vi "Alpha_Beta_prunning.vi"(0 "Game":i32[][](array[numeric]), 1 "Active Turn":i32=1, 2 "Depth":i32, 5 "NextTurn":i32=1) -> (10 "Win":bool, 11 "GameOver":bool, 14 "Score":i32, 15 "Next Move":cluster{"Row":i32, "Col":i32}, 17 "Scores":i32[](array[numeric]), 18 "Moves":cluster{"Row":i32, "Col":i32}[](array[cluster]))   [LabVIEW 2017]
panel:
  out "Array (Ausgang)":i32[][](array[numeric])
  in  "Max Depth (7)":i32=7 min=7 max=23
  # "3x3 Felder Max Depth 7\n4*4 Felder Max Depth 15\n5*5 Felder Max Depth 23"
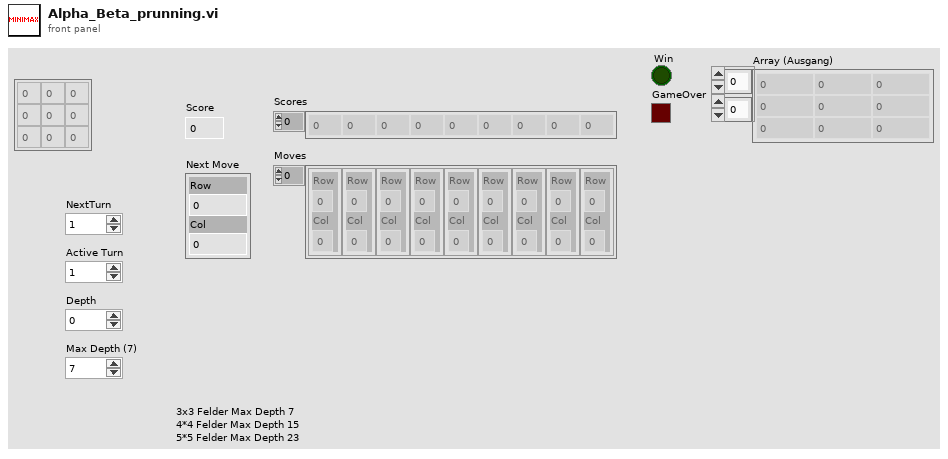
[diagram p1: front panel]
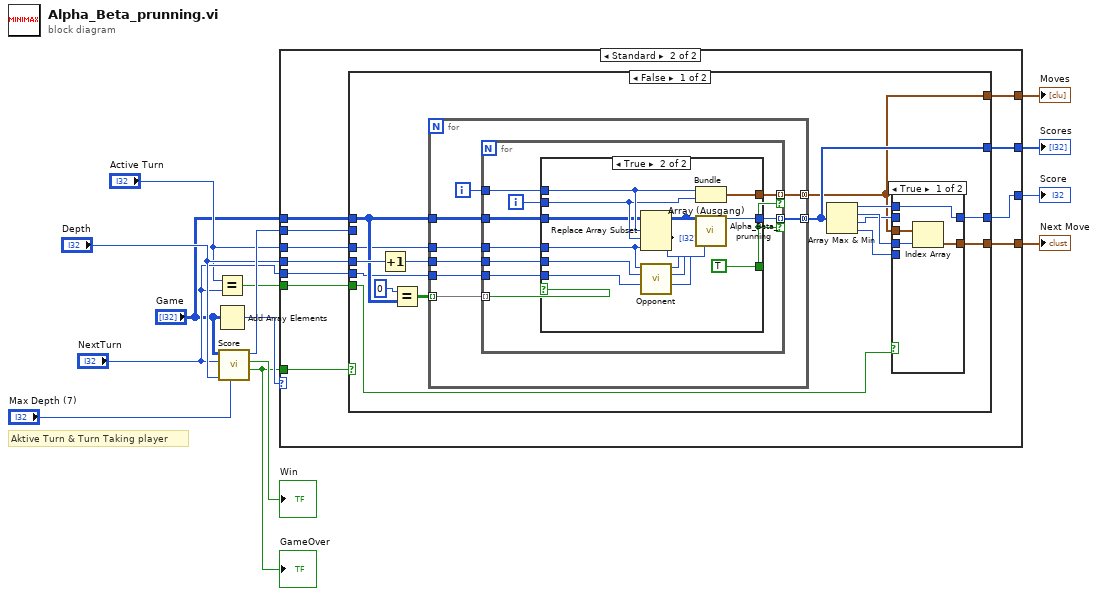
[diagram p0: block diagram]
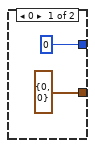
[diagram p2: hidden frame]
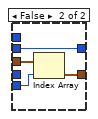
[diagram p3: hidden frame]
diagram:
  # "Aktive Turn & Turn Taking player"
  n1 = Equal?(x="Active Turn", y="NextTurn") -> (x = y?=w9:bool)
  n2 = Add Array Elements(numeric array="Game") -> (sum=w4:i32)
  n3 = call "Score.vi"("Max Depth (8)"="Max Depth (7)", "Depth"="Depth", "Turn Taking Player"="NextTurn", "Game"="Game") -> ("Game over"=w1:bool, "Win"=→"Win":bool, "Score"=w13:i32)  [unwired: 5 in]
  "GameOver" <- w1
  n4 = case shown="Standard" w4 {
    tunnel: [0 ("Score") w27] -> w14
    tunnel: w13 -> [_ w26]
    tunnel: [cluster{"Row":i32, "Col":i32} {"Row"=0, "Col"=0} ("Move") w25] -> w12
    tunnel: [_ w24] -> w11
    tunnel: [_ w23] -> w10
    tunnel: w9 -> [_ w22]
    tunnel: "Depth" -> [_ w21]
    tunnel: "NextTurn" -> [_ w20]
    tunnel: "Active Turn" -> [_ w19]
    tunnel: w1 -> [_ w18]
    tunnel: "Game" -> [_ w17]
    frame 0 {
    }
    frame Default {
      n5 = case shown="False" w18 {
        tunnel: [w34 w81] -> w27
        tunnel: w26 -> [_ w81]
        tunnel: w21 -> [w43 _]
        tunnel: w17 -> [w40 _]
        tunnel: w19 -> [w38 _]
        tunnel: [w35 _] -> w25
        tunnel: [w31 _] -> w23
        tunnel: [w30 _] -> w24
        tunnel: w20 -> [w29 _]
        tunnel: w22 -> [w28 _]
        frame False {
          n6 = Increment(x=w43) -> (x+1=w39:i32)
          n7 = Equal?(x=0, y=w40) -> (x = y?=w41:bool[][])
          n8 = for {
            tunnel: w41 -> [w59] mode=indexing
            tunnel: w40 -> [w57]
            tunnel: w39 -> [w56]
            tunnel: w38 -> [w53]
            tunnel: w29 -> [w52]
            tunnel: [w55] -> w31 mode=concatenating
            tunnel: [w54] -> w30 mode=concatenating
            i -> [w58]
            n9 = for {
              tunnel: w59 -> [w69] mode=indexing
              tunnel: w58 -> [w67]
              tunnel: w57 -> [w68]
              tunnel: w56 -> [w65]
              tunnel: w53 -> [w62]
              tunnel: w52 -> [w61]
              tunnel: [w64] -> w55 mode=indexing if=w60
              tunnel: [w63] -> w54 mode=indexing if=w60
              i -> [w66]
              n10 = case shown="True" w69 {
                tunnel: w68 -> [_ w70]
                tunnel: w67 -> [_ w78]
                tunnel: w66 -> [_ w77]
                tunnel: w65 -> [_ w79]
                tunnel: [_ w73] -> w64
                tunnel: [_ w72] -> w63
                tunnel: w62 -> [_ w75]
                tunnel: w61 -> [_ w76]
                tunnel: [_ TRUE] -> w60
                frame False {
                }
                frame True {
                  n11 = Replace Array Subset(array=w70, new element=w75, index (row)=w78, index (col)=w77) -> (w80:i32[][])
                  "Array (Ausgang)" <- w80
                  n12 = call "Opponent.vi"("Player"=w75) -> ("Opponent"=w74:i32)  [unwired: 10 in]
                  n13 = Bundle(w78, w77) -> (w72:cluster{i32, i32})  [unwired: 1 in]
                  n14 = call "Alpha_Beta_prunning.vi"("Game"=w80, "Active Turn"=w74, "Depth"=w79, "NextTurn"=w76) -> ("Score"=w73:i32)  [unwired: 10 in, 5 out]
                }
              }
            }
          }
          n15 = Array Max & Min(array=w31) -> (max value=w33:i32, max index (indices)=w37:i32, min value=w32:i32, min index (indices)=w36:i32)
          n16 = case shown="True" w28 {
            tunnel: w30 -> [w47 w51]
            tunnel: w37 -> [w44 _]
            tunnel: w36 -> [_ w48]
            tunnel: [w46 w50] -> w35
            tunnel: [w45 w49] -> w34
            tunnel: w33 -> [w45 _]
            tunnel: w32 -> [_ w49]
            frame True {
              n17 = Index Array(array=w47, index=w44) -> (element=w46:cluster{i32, i32})
            }
            frame False {
              n18 = Index Array(array=w51, index=w48) -> (element=w50:cluster{i32, i32})
            }
          }
        }
        frame True {
        }
      }
    }
  }
  "Score" <- w14
  "Next Move" <- w12
  "Scores" <- w10
  "Moves" <- w11
